vi "BASE_Reporting.vi"(8 "error in (no error)":errorcluster) -> (0 "error out":errorcluster)   [LabVIEW 2017]
uses:
  <vilib>/Utility/miscctls.llb/LVRowAndColumnTypeDef.ctl
  <vilib>/addons/database/Connection.llb/DB Tools Open Connec (Path).vi
  <vilib>/Utility/file.llb/Write Delimited Spreadsheet (string).vi
  <vilib>/addons/database/NI_Database_API.lvlib
panel:
  in  "FROM DATE 2":timestamp format="%<%d/%m/%Y>T"
  in  "TO DATE  2":timestamp format="%<%d/%m/%Y>T"
  out "Data History Table":string[][](table)
  out "Selection Start":T1
  in  "Show Report":bool
  in  "Export to Excel":bool
  in  "Delete Button":bool
  in  "Machine Selection":string(combo)="ALL STATION"
  out "From Date":string
  out "appended path":path
  in  "SELECT FILTER":string(combo)="PART_NO"
  out "DESCRIPTION":string
  in  "TO DATE":timestamp format="%<%d/%m/%Y>T"
  in  "FROM DATE":timestamp format="%<%d/%m/%Y>T"
  in  "Back":bool
  # "BARCODE VERIFICATION SYSTEM REPORTS"
  # "Data History Table"
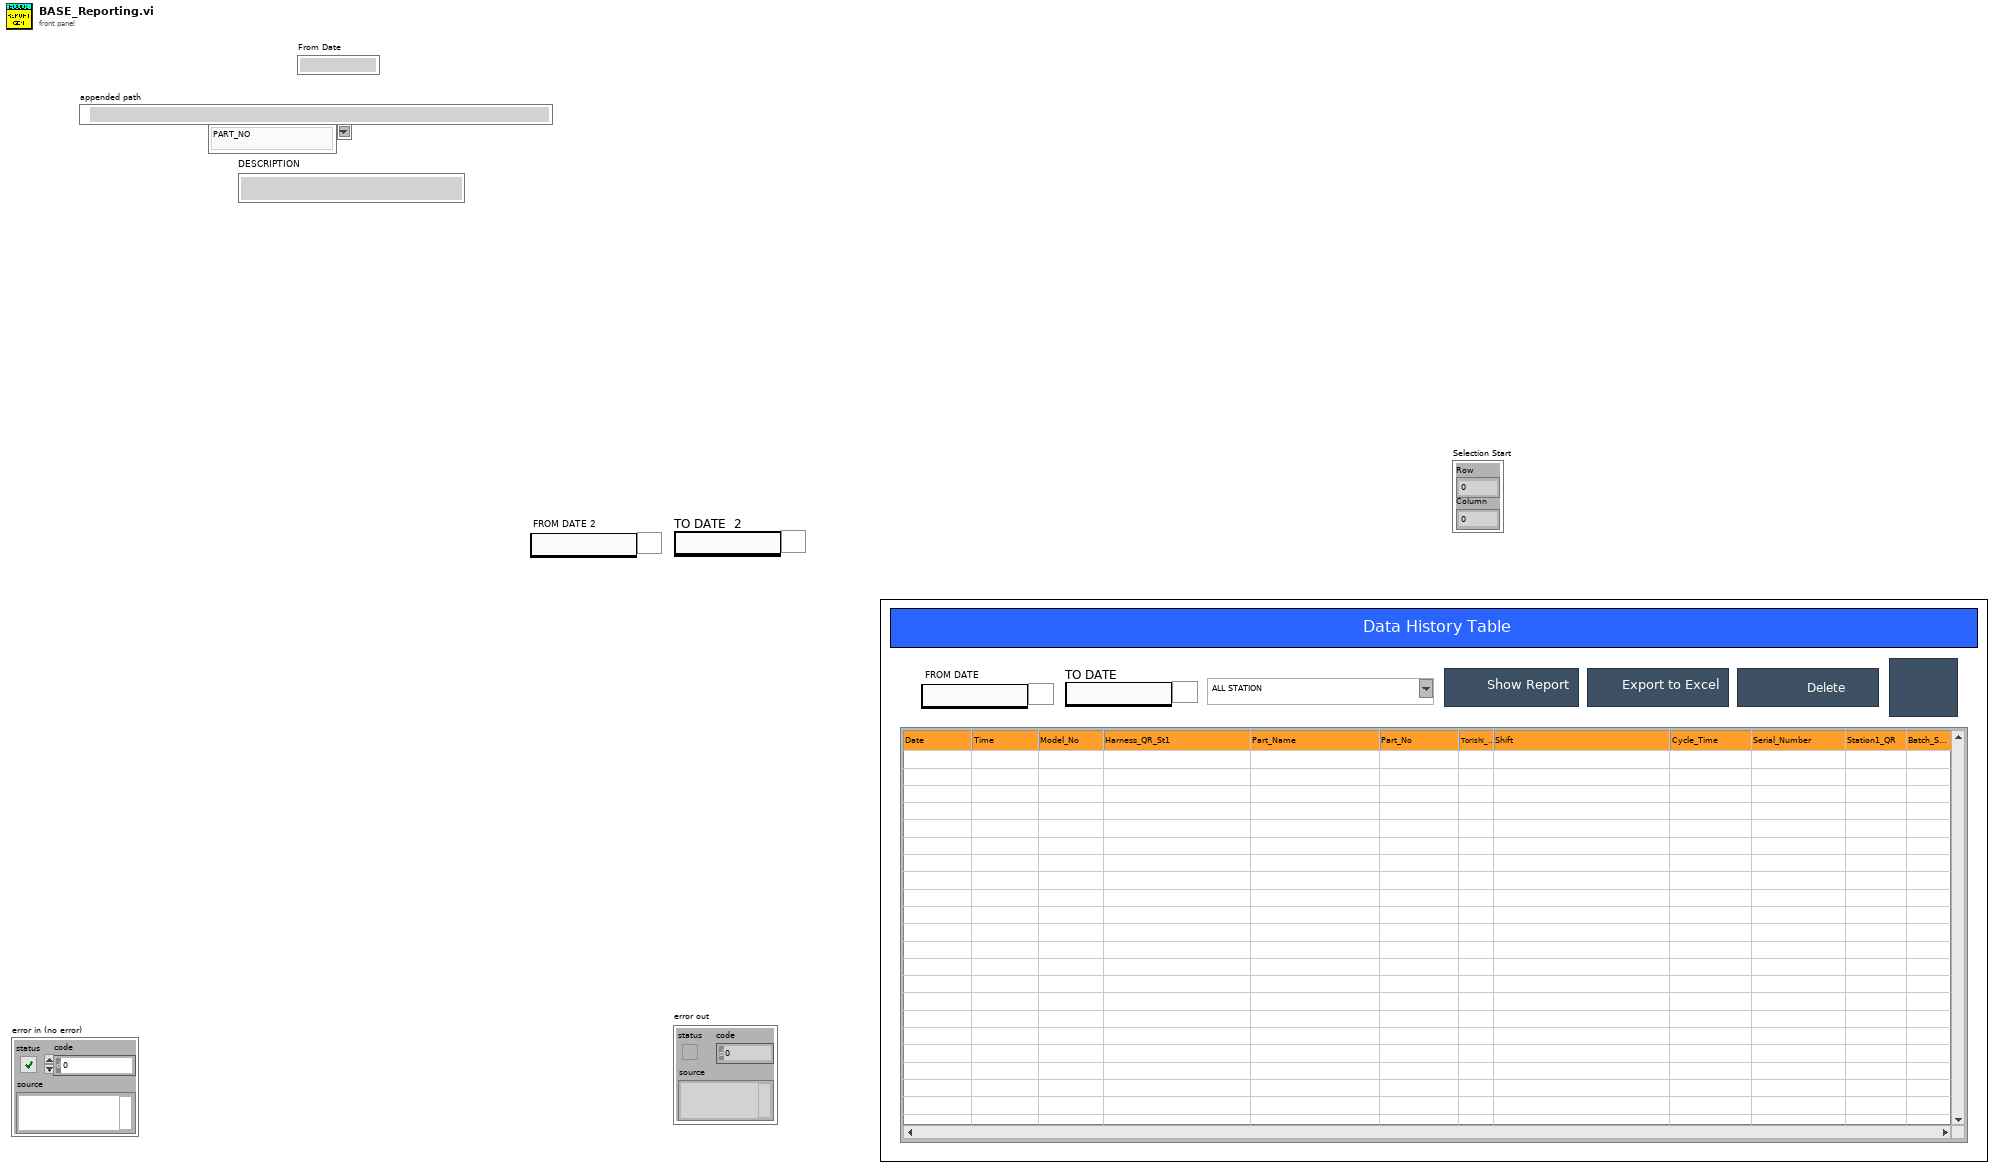
[diagram p1: front panel]
types:
  T1 = typedef "LVRowAndColumnTypeDef.ctl" = cluster{"Row":i32, "Column":i32}
  T2 = enum8{"Enabled", "Disabled", "Disabled and Grayed Out"}
  T3 = typedef "NI_Database_API.lvlib/Conn ObjectReference.ctl" = refnum<k1>
  T4 = enum32{"Invalid", "Standard", "Closed", "Hidden", "Minimized", "Maximized"}
  T5 = enum32{"invalid app kind", "Development System", "Run Time System", "Student Edition", "Embedded LabVIEW", "Evaluation", "Custom"}
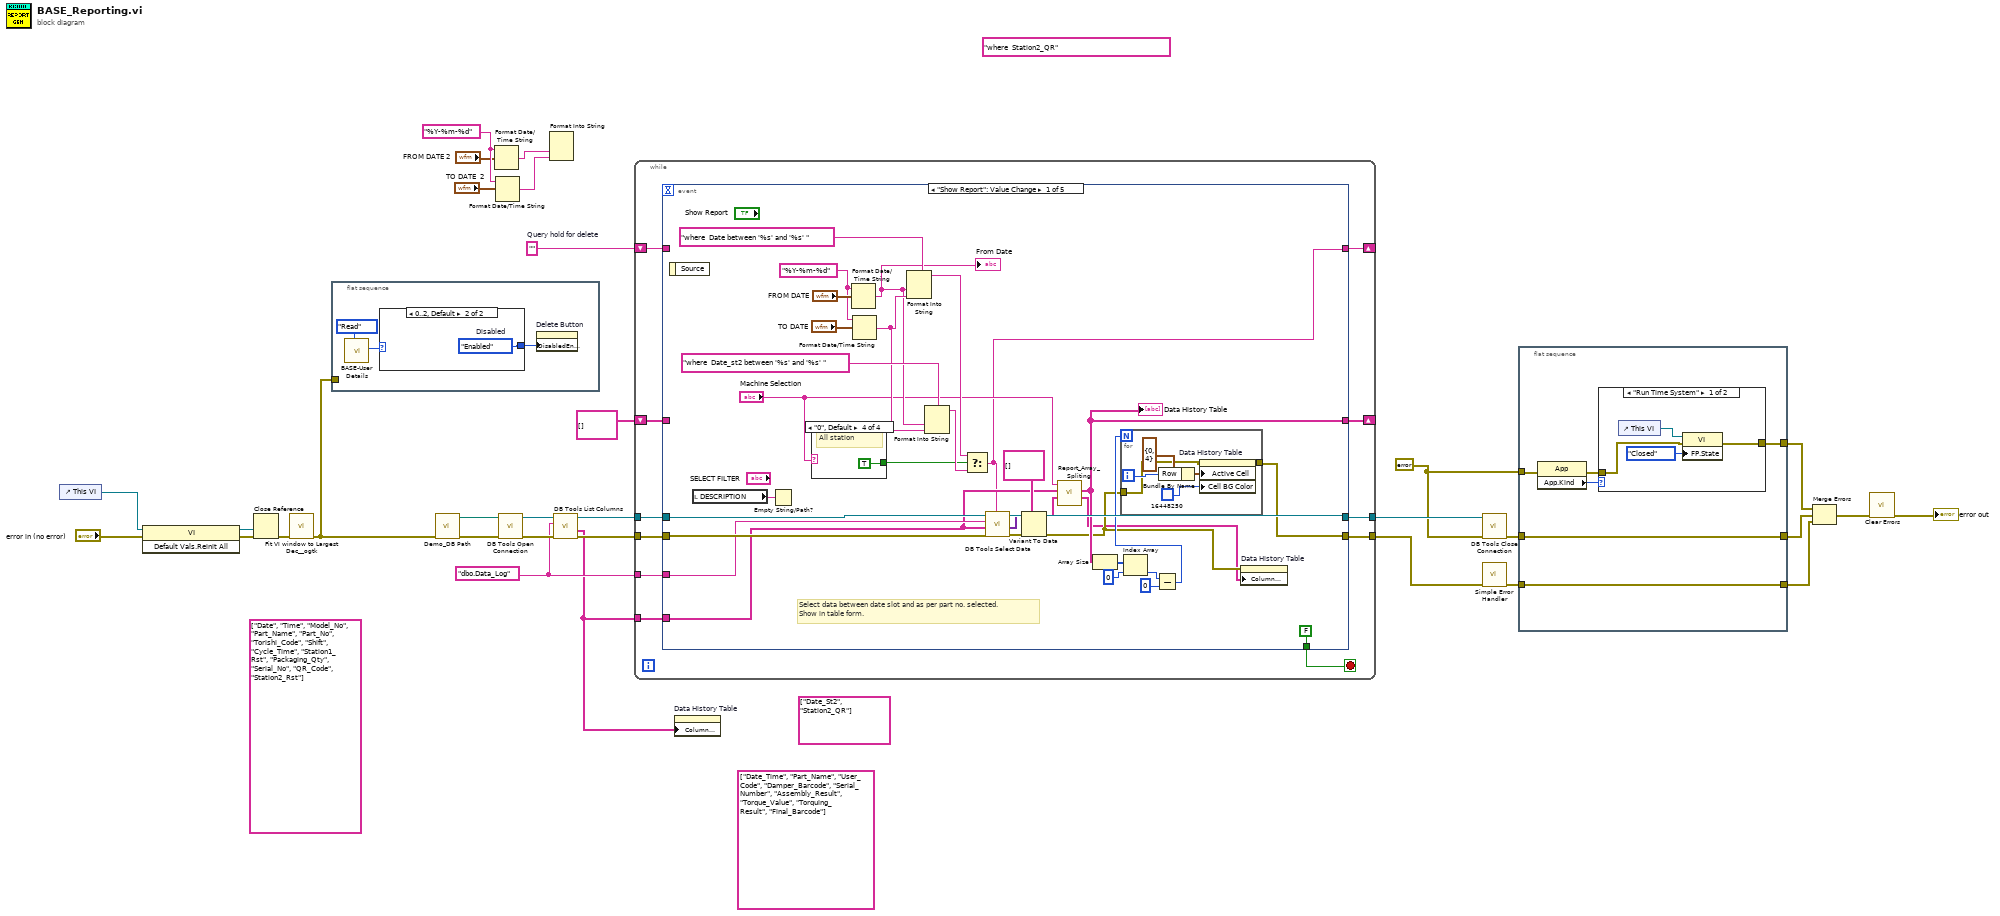
[diagram p0: block diagram]
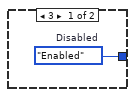
[diagram p2: hidden frame]
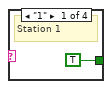
[diagram p4: hidden frame]
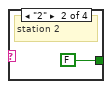
[diagram p5: hidden frame]
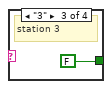
[diagram p6: hidden frame]
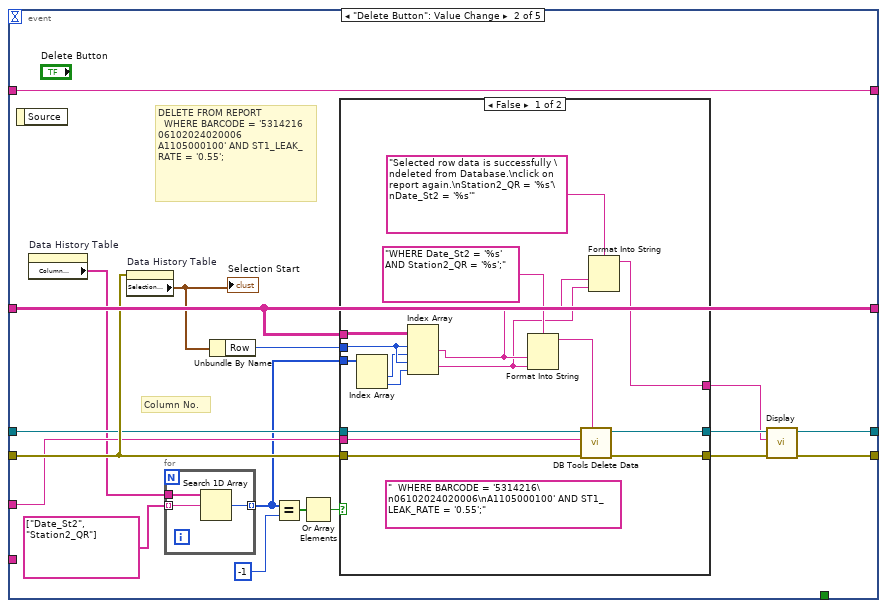
[diagram p7: hidden frame]
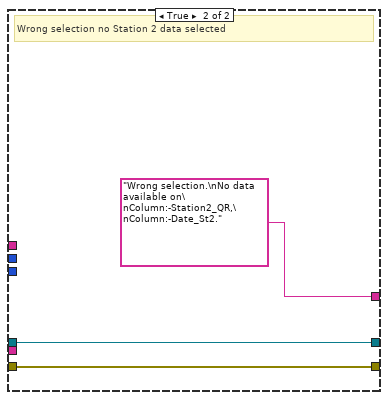
[diagram p8: hidden frame]
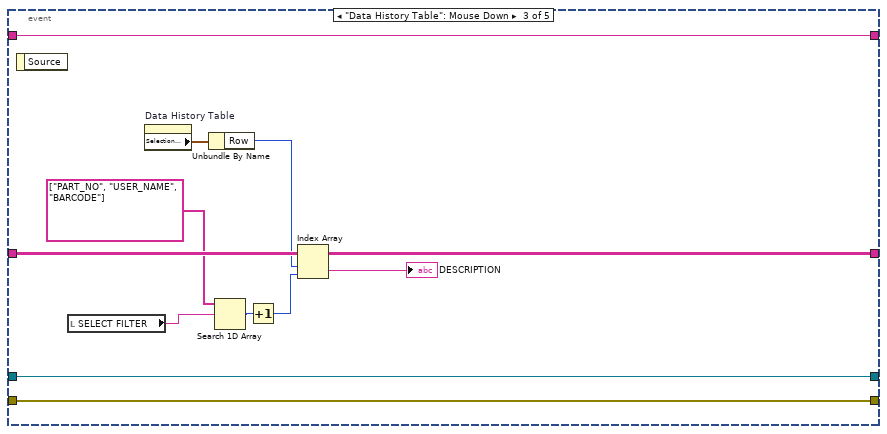
[diagram p9: hidden frame]
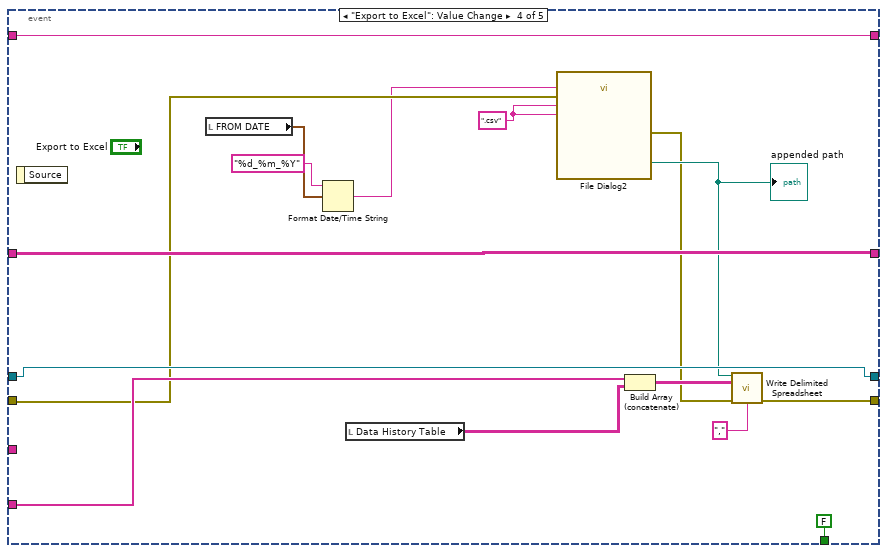
[diagram p10: hidden frame]
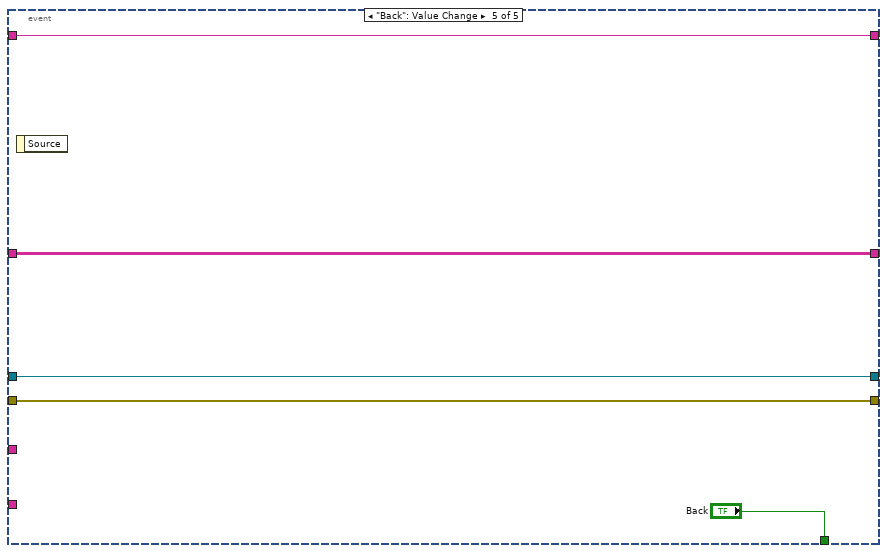
[diagram p11: hidden frame]
diagram:
  (unwired) string[] ["Date_St2", "Station2_QR"]
  w3 = "%Y-%m-%d"
  (unwired) "where  Station2_QR" ("format string")
  w6 = ""  # Query hold for delete
  (unwired) string[] ["Date", "Time", "Model_No", "Part_Name", "Part_No", "Torishi_Code", "Shift", "Cycle_Time", "Station1_Rst", "Packaging_Qty", "Serial_No", "QR_Code", "Station2_Rst"] ("columns 2")
  w9 = "dbo.Data_Log" ("table")
  (unwired) string[] ["Date_Time", "Part_Name", "User_Code", "Damper_Barcode", "Serial_Number", "Assembly_Result", "Torque_Value", "Torquing_Result", "Final_Barcode"]
  w26 = errorcluster {"status"=FALSE, "code"=0, "source"=""} ("error in (no error)")
  n1 = control-ref of="This VI"() -> (w20:refnum<vi>)
  n2 = invoke class="VI" method="Default Vals.Reinit All"(reference=w20, error in="error in (no error)") -> (reference out=w18:refnum<vi>, error out=w17:errorcluster)  [unwired: 1 in, 1 out]
  n3 = Close Reference(reference=w18, error in (no error)=w17) -> (error out=w16:errorcluster)
  n4 = call <userlib>:"Fit VI window to Largest Dec__ogtk.vi"("error in (no error)"=w16) -> ("error out"=w7:errorcluster)  [unwired: 5 in, 1 out]
  n5 = flat-sequence {
    tunnel: w7 -> [_]
    frame #0 {
      n6 = call "BASE-User Details.vi"("Enum"=enum16{"Read", "Write"}."Read") -> ("Level Out"=w33:i32)  [unwired: 9 in, 1 out]
      n7 = case shown="0..2, Default" w33 {
        tunnel: [w35 w36] -> w32
        frame 3 {
          w35 = T2."Enabled"  # Disabled
        }
        frame 0..2, Default {
          w36 = T2."Enabled"  # Disabled
        }
      }
      n8 = property on="Delete Button" class="Bool"("DisabledEnum"=w32) -> ()  [unwired: 2 in, 2 out]
    }
  }
  n9 = call "Demo_DB Path.vi"("error in"=w7) -> ("error out"=w15:errorcluster, "DB Path"=w14:path)  [unwired: 9 in]
  n10 = Format Date/Time String(time format string (%c)=w3, seconds (now)="FROM DATE 2") -> (date/time string=w5:string)  [unwired: 1 in]
  n11 = Format Date/Time String(time format string (%c)=w3, seconds (now)="TO DATE  2") -> (date/time string=w4:string)  [unwired: 1 in]
  n12 = call-poly <vilib>:"DB Tools Open Connection.vi"("error in (no error)"=w15, "connection information"=w14) -> ("error out"=w13:errorcluster, "connection reference"=w11:T3)  [unwired: 6 in]
  n13 = Format Into String(w5, w4) -> ()  [unwired: 3 in, 2 out]
  n14 = call <vilib>:"DB Tools List Columns.vi"("error in (no error)"=w13, "table"=w9, "connection reference"=w11) -> ("error out"=w12:errorcluster, "columns"=w8:string[], "connection reference out"=w10:T3)  [unwired: 1 in, 1 out]
  n15 = while {
    tunnel: w8 -> [w43]
    tunnel: w9 -> [w42]
    tunnel: w10 -> [w47]
    tunnel: [w44] -> w31
    tunnel: w12 -> [w46]
    tunnel: [w45] -> w29
    shift-right: [w40] -> _
    shift-left: string[][] [] -> [w39]
    shift-right: [w38] -> _
    shift-left: w6 -> [w37]
    stop <- w41 stop-if-true
    n16 = event shown="[0] \"Show Report\": Value Change" {
      selector: _ -> [_ _ _ _ _]
      dyn-events: _ -> [_ _ _ _ _]
      timeout: _ -> [_ _ _ _ _]
      tunnel: w47 -> [w79 w102 w136 w155 w159]
      tunnel: w46 -> [w78 w103 w135 w146 w158]
      tunnel: [w62 w91 w135 w150 w158] -> w45
      tunnel: [w77 w101 w136 w155 w159] -> w44
      tunnel: w43 -> [w56 _ _ w151 _]
      tunnel: w42 -> [w76 w100 _ _ _]
      tunnel: [FALSE ("Back") _ _ FALSE ("Back") "Back"] -> w41
      tunnel: [w58 w105 w139 w152 w157] -> w40
      tunnel: w39 -> [_ w105 w139 w152 w157]
      tunnel: [w48 w106 w129 w140 w156] -> w38
      tunnel: w37 -> [_ w106 w129 w140 w156]
      event "Show Report": Value Change {
        w66 = "%Y-%m-%d"
        # "Select data between date slot and as per part no. selected.\nShow in table form."
        n17 = event-data() -> ()  [unwired: 1 in, 1 out]
        n18 = local read "DESCRIPTION"() -> (w65:string)
        n19 = Empty String/Path?(string/path=w65) -> ()  [unwired: 1 out]
        n20 = case shown="\"0\", Default" "Machine Selection" {
          tunnel: [TRUE FALSE FALSE TRUE] -> w49
          frame "1" {
            # "Station 1"
          }
          frame "2" {
            # "station 2"
          }
          frame "3" {
            # "station 3"
          }
          frame "0", Default {
            # "All station"
          }
        }
        n21 = Format Date/Time String(time format string (%c)=w66, seconds (now)="FROM DATE") -> (date/time string=w51:string)  [unwired: 1 in]
        "From Date" <- w51
        n22 = Format Date/Time String(time format string (%c)=w66, seconds (now)="TO DATE") -> (date/time string=w52:string)  [unwired: 1 in]
        n23 = Format Into String(format string="where  Date between '%s' and '%s' ", w51, w52) -> (resulting string=w70:string)  [unwired: 2 in, 1 out]
        n24 = Format Into String(format string="where  Date_st2 between '%s' and '%s' ", w51, w52) -> (resulting string=w71:string)  [unwired: 2 in, 1 out]
        n25 = Select(t=w70, s=w49, f=w71) -> (s? t:f=w48:string)
        n26 = call <vilib>:"DB Tools Select Data.vi"("condition"=w48, "error in (no error)"=w78, "columns"=w56, "table"=w76, "connection reference"=w79) -> ("error out"=w72:errorcluster, "data"=w75:variant[][], "connection reference out"=w77:T3)  [unwired: 1 in]
        n27 = Variant To Data(error in=w72, type=string[][] [], Variant=w75) -> (data=w57:string[][], error out=w55:errorcluster)
        n28 = call "Report_Array_Spliting.vi"("Input array 2"=w57, "columns Header"=w56, "Machine Selection"="Machine Selection") -> ("collumns Header out"=w54:string[], "Output"=w58:string[][])  [unwired: 6 in]
        "Data History Table" <- w58
        n29 = Array Size(array=w58) -> (size(s)=w64:i32[])
        n30 = Index Array(array=w64, index=0) -> (element=w60:i32)
        n31 = Subtract(x=w60, y=0) -> (x-y=w59:i32)
        n32 = for {
          N: w59 -> [_]
          tunnel: w55 -> [w85]
          tunnel: [w84] -> w62
          i -> [w87]
          n33 = Bundle By Name(cluster=T1 {"Row"=0, "Column"=4} ("Active Cell:Active Cell"), "Row"=w87) -> (w88:T1)
          n34 = property on="Data History Table" class="Tbl (strict)"(error in=w85, "Active Cell"=w88, "Cell BG Color"=u32 16448250) -> (error out=w84:errorcluster)  [unwired: 1 in, 1 out]
        }
        n35 = property on="Data History Table" class="Tbl (strict)"(error in=w55, "Column Headers[]"=w54) -> ()  [unwired: 1 in, 2 out]
      }
      event "Delete Button": Value Change {
        # "Column No."
        # "DELETE FROM REPORT\n  WHERE BARCODE = '5314216\n06102024020006\nA1105000100' AND ST1_LEAK_RATE = '0.55';"
        n36 = event-data() -> ()  [unwired: 1 in, 1 out]
        n37 = property on="Data History Table" class="Tbl (strict)"() -> ("Column Headers[]"=w99:string[])  [unwired: 2 in, 2 out]
        n38 = property on="Data History Table" class="Tbl (strict)"(error in=w103) -> ("Selection Start"=w104:T1)  [unwired: 1 in, 2 out]
        "Selection Start" <- w104
        n39 = for {
          tunnel: w99 -> [w128]
          tunnel: string[] ["Date_St2", "Station2_QR"] -> [w127] mode=indexing
          tunnel: [w126] -> w93 mode=indexing
          n40 = Search 1D Array(1D array=w128, element=w127) -> (index of element=w126:i32)  [unwired: 1 in]
        }
        n41 = Unbundle By Name(w104) -> ("Row"=w97:i32)
        n42 = Equal?(x=w93, y=-1 ("index of element")) -> (x = y?=w95:bool[])
        n43 = Or Array Elements(Boolean array=w95) -> (logical OR=w94:bool)
        n44 = case shown="False" w94 {
          tunnel: w105 -> [w122 _]
          tunnel: w103 -> [w121 w125]
          tunnel: [w120 w125] -> w92
          tunnel: w102 -> [w119 w124]
          tunnel: [w118 w124] -> w101
          tunnel: w100 -> [w117 _]
          tunnel: w97 -> [w116 _]
          tunnel: w93 -> [w115 _]
          tunnel: [w107 "Wrong selection.\nNo data available on\nColumn:-Station2_QR,\nColumn:-Date_St2."] -> w90
          frame False {
            (unwired) "  WHERE BARCODE = '5314216\n06102024020006\nA1105000100' AND ST1_LEAK_RATE = '0.55';"
            n45 = Index Array(array=w115) -> (element #1=w114:i32, element #2=w113:i32)  [unwired: 2 in]
            n46 = Index Array(array=w122, index (row) #1=w116, index (col) #1=w114, index (row) #2=w116, index (col) #2=w113) -> (element #1=w110:string, element #2=w109:string)
            n47 = Format Into String(format string="WHERE Date_St2 = '%s' AND Station2_QR = '%s';", w110, w109) -> (resulting string=w111:string)  [unwired: 2 in, 1 out]
            n48 = call <vilib>:"DB Tools Delete Data.vi"("condition"=w111, "error in (no error)"=w121, "table"=w117, "connection reference"=w119) -> ("error out"=w120:errorcluster, "connection reference out"=w118:T3)  [unwired: 6 in]
            n49 = Format Into String(format string="Selected row data is successfully \ndeleted from Database.\nclick on report again.\nStation2_QR = '%s'\nDate_St2 = '%s'", w110, w109) -> (resulting string=w107:string)  [unwired: 2 in, 1 out]
          }
          frame True {
            # "Wrong selection no Station 2 data selected"
          }
        }
        n50 = call "Display"("error in (no error)"=w92, "Message"=w90) -> ("error out"=w91:errorcluster)  [unwired: 8 in, 1 out]
      }
      event "Data History Table": Mouse Down {
        n51 = event-data() -> ()  [unwired: 1 in, 1 out]
        n52 = local read "SELECT FILTER"() -> (w132:string)
        n53 = property on="Data History Table" class="Tbl (strict)"() -> ("Selection Start"=w138:T1)  [unwired: 2 in, 2 out]
        n54 = Unbundle By Name(w138) -> ("Row"=w137:i32)
        n55 = Search 1D Array(1D array=string[] ["PART_NO", "USER_NAME", "BARCODE"], element=w132) -> (index of element=w131:i32)  [unwired: 1 in]
        n56 = Increment(x=w131) -> (x+1=w130:i32)
        n57 = Index Array(array=w139, index (row)=w137, index (col)=w130) -> (element=→"DESCRIPTION":string)
      }
      event "Export to Excel": Value Change {
        w149 = ".csv" ("pattern label")
        n58 = event-data() -> ()  [unwired: 1 in, 1 out]
        n59 = local read "FROM DATE"() -> (w144:timestamp)
        n60 = Format Date/Time String(time format string (%c)="%d_%m_%Y", seconds (now)=w144) -> (date/time string=w143:string)  [unwired: 1 in]
        n61 = local read "Data History Table"() -> (w141:string[][])
        n62 = call "File Dialog2"("default name"=w143, "error in"=w146, "pattern (all files)"=w149, "pattern label"=w149) -> ("selected path"=w148:path, "error out"=w147:errorcluster)  [unwired: 8 in, 2 out]
        "appended path" <- w148
        n63 = Build Array (concatenate)(w151, w141) -> (w153:string[][])
        n64 = call-poly <vilib>:"Write Delimited Spreadsheet.vi"("file path (dialog if empty)"=w148, "2D data"=w153, "error in (no error)"=w147, "delimiter (\\t)"="," ("delimiter (\\t)")) -> ("error out"=w150:errorcluster)  [unwired: 10 in, 1 out]
      }
      event "Back": Value Change {
        n65 = event-data() -> ()  [unwired: 1 in, 1 out]
      }
    }
  }
  n66 = property on="Data History Table" class="Tbl (strict)"("Column Headers[]"=w8) -> ()  [unwired: 2 in, 2 out]
  n67 = call <vilib>:"DB Tools Close Connection.vi"("error in (no error)"=w26, "connection reference"=w31) -> ("error out"=w24:errorcluster)  [unwired: 5 in]
  n68 = call <vilib>:"Simple Error Handler.vi"("error in (no error)"=w29) -> ("error out"=w22:errorcluster)  [unwired: 4 in, 4 out]
  n69 = flat-sequence {
    tunnel: [w164] -> w27
    tunnel: w26 -> [w163]
    tunnel: [w162] -> w25
    tunnel: w24 -> [w162]
    tunnel: [w161] -> w23
    tunnel: w22 -> [w161]
    frame #0 {
      n70 = property class="App"(error in=w163) -> (error out=w165:errorcluster, "App.Kind"=w166:T5)  [unwired: 1 in, 1 out]
      n71 = case shown="\"Run Time System\"" w166 {
        tunnel: w165 -> [w168 w171]
        tunnel: [w167 w171] -> w164
        frame "Run Time System" {
          n72 = control-ref of="This VI"() -> (w170:refnum<vi>)
          n73 = property class="VI"(reference=w170, error in=w168, "FP.State"=T4."Closed" ("Front Panel Window:State")) -> (error out=w167:errorcluster)  [unwired: 1 out]
        }
        frame "Development System", Default {
        }
      }
    }
  }
  n74 = Merge Errors(w27, w25, w23) -> (w28:errorcluster)
  n75 = call <vilib>:"Clear Errors.vi"("error in (no error)"=w28) -> ("error out"=→"error out":errorcluster)  [unwired: 5 in, 1 out]
